vi "Vision Processing.vi"(7 "Image Size":T1=enum."320x240", 11 "error in":errorcluster) -> (4 "Sorted Scores":T6(array[cluster]) {"Correlation" format="%#_3g"; "Scale %" format="%#_3g"; "Score" format="%#_3g"}, 6 "Detected Totes":T7(array[cluster]) {"Normalized Rect"."Numeric 5" format="%#_2g"; "Normalized Rect"."Numeric 3" format="%#_2g"; "Normalized Rect"."Numeric 2" format="%#_2g"; "Normalized Rect"."Numeric" format="%#_2g"}, 8 "Particles":i32, 10 "ms to process":u32, 15 "error out":errorcluster)   [LabVIEW 2014]
doc: "This VI runs in parallel to other tasks. It gets images from the camera, processes them for color or shape and use that information to affect robot behavior."
uses:
  <vilib>/Rock Robotics/WPI/Camera/WPI_CameraSettings Read MJPG.ctl
  <vilib>/Rock Robotics/WPI/Camera/WPI_CameraImageSize.ctl
  2015-Vision/Vision/Users/Jarren/Desktop/Vision Support Code/Camera Types.ctl
  <vilib>/vision/Pattern Matching.llb/IMAQ Match Range Setting.ctl
  <vilib>/vision/Pattern Matching.llb/IMAQ Curve Parameters.ctl
  <vilib>/vision/NI_Vision_Development_Module.lvlib
panel:
  out "error out 2":errorcluster
  in  "Image Size 2":T1=enum."320x240"
  in  "error in 2":errorcluster
  out "Masked 2":T2(plugin-control)
  in  "Tote Color 2":T3={"Hue"={23.67058792990901, 48.923317529462665}, "Sat"={66.78571428571429, 255.0}, "Val"={48.571428571428584, 255.0}} {"Hue" scale=0.0..255.0 scale format="%#_3g"}
  out "Particles 2":i32
  out "ms to process 2":u32
  in  "Source 2":enum32{"Files", "Camera"}(tab)
  in  "Images 2":i32(listbox)
  in  "Folder Location 2":path=path "Sample Images/KicoffFilmingVision"
  in  "Camera Settings 2":T4={"fps"=20, "compression"=30, "Image Size"=enum."320x240"}
  in  "Camera Address 2":string="USB 1"
  in  "image files 2":string[](array[string])
  in  "Image Path 2":path=path "Sample Images/KicoffFilmingVision"
  in  "Camera Type 2":T5=enum."MS HD3000 square"
  out "Original Image 2":T2(plugin-control)
  out "Template 2":T2(plugin-control)
  out "Sorted Scores 2":T6(array[cluster]) {"Correlation" format="%#_3g"; "Scale %" format="%#_3g"; "Score" format="%#_3g"}
  in  "Annotate 2":bool=TRUE
  in  "Score Threshold 2":dbl=75.0
  out "Detected Totes 2":T7(array[cluster]) {"Normalized Rect"."Numeric 5" format="%#_2g"; "Normalized Rect"."Numeric 3" format="%#_2g"; "Normalized Rect"."Numeric 2" format="%#_2g"; "Normalized Rect"."Numeric" format="%#_2g"}
  out "Template":T2(plugin-control)
  in  "Camera Type":T5=enum."MS HD3000 square"
  in  "Image Path":path=path "Sample Images/KicoffFilmingVision"
  in  "image files":string[](array[string])
  in  "Score Threshold":dbl=75.0
  in  "Source":enum32{"Files", "Camera"}(tab)
  in  "Images":i32(listbox)
  in  "Folder Location":path=path "Sample Images/KicoffFilmingVision"
  in  "Camera Settings":T4={"fps"=20, "compression"=30, "Image Size"=enum."320x240"}
  in  "Camera Address":string="USB 1"
  in  "Annotate":bool=TRUE
  in  "Tote Color":T3={"Hue"={23.67058792990901, 48.923317529462665}, "Sat"={66.78571428571429, 255.0}, "Val"={48.571428571428584, 255.0}} {"Hue" scale=0.0..255.0 scale format="%#_3g"}
  out "Masked":T2(plugin-control)
  out "Original Image":T2(plugin-control)
  # "Instructions:\nUse Source to select image files from a directory or use a USB or IP camera connected to your laptop.\nUse Tote Color for initial processing, then search for the trained template image. Use Vision Assistant\nto train for different images or to modify Range Settings. \nThis example is effective within a few feet. It is likely not the right choice for distant patterns.\nAnnotations show the rectangle and the scores from top to bottom."
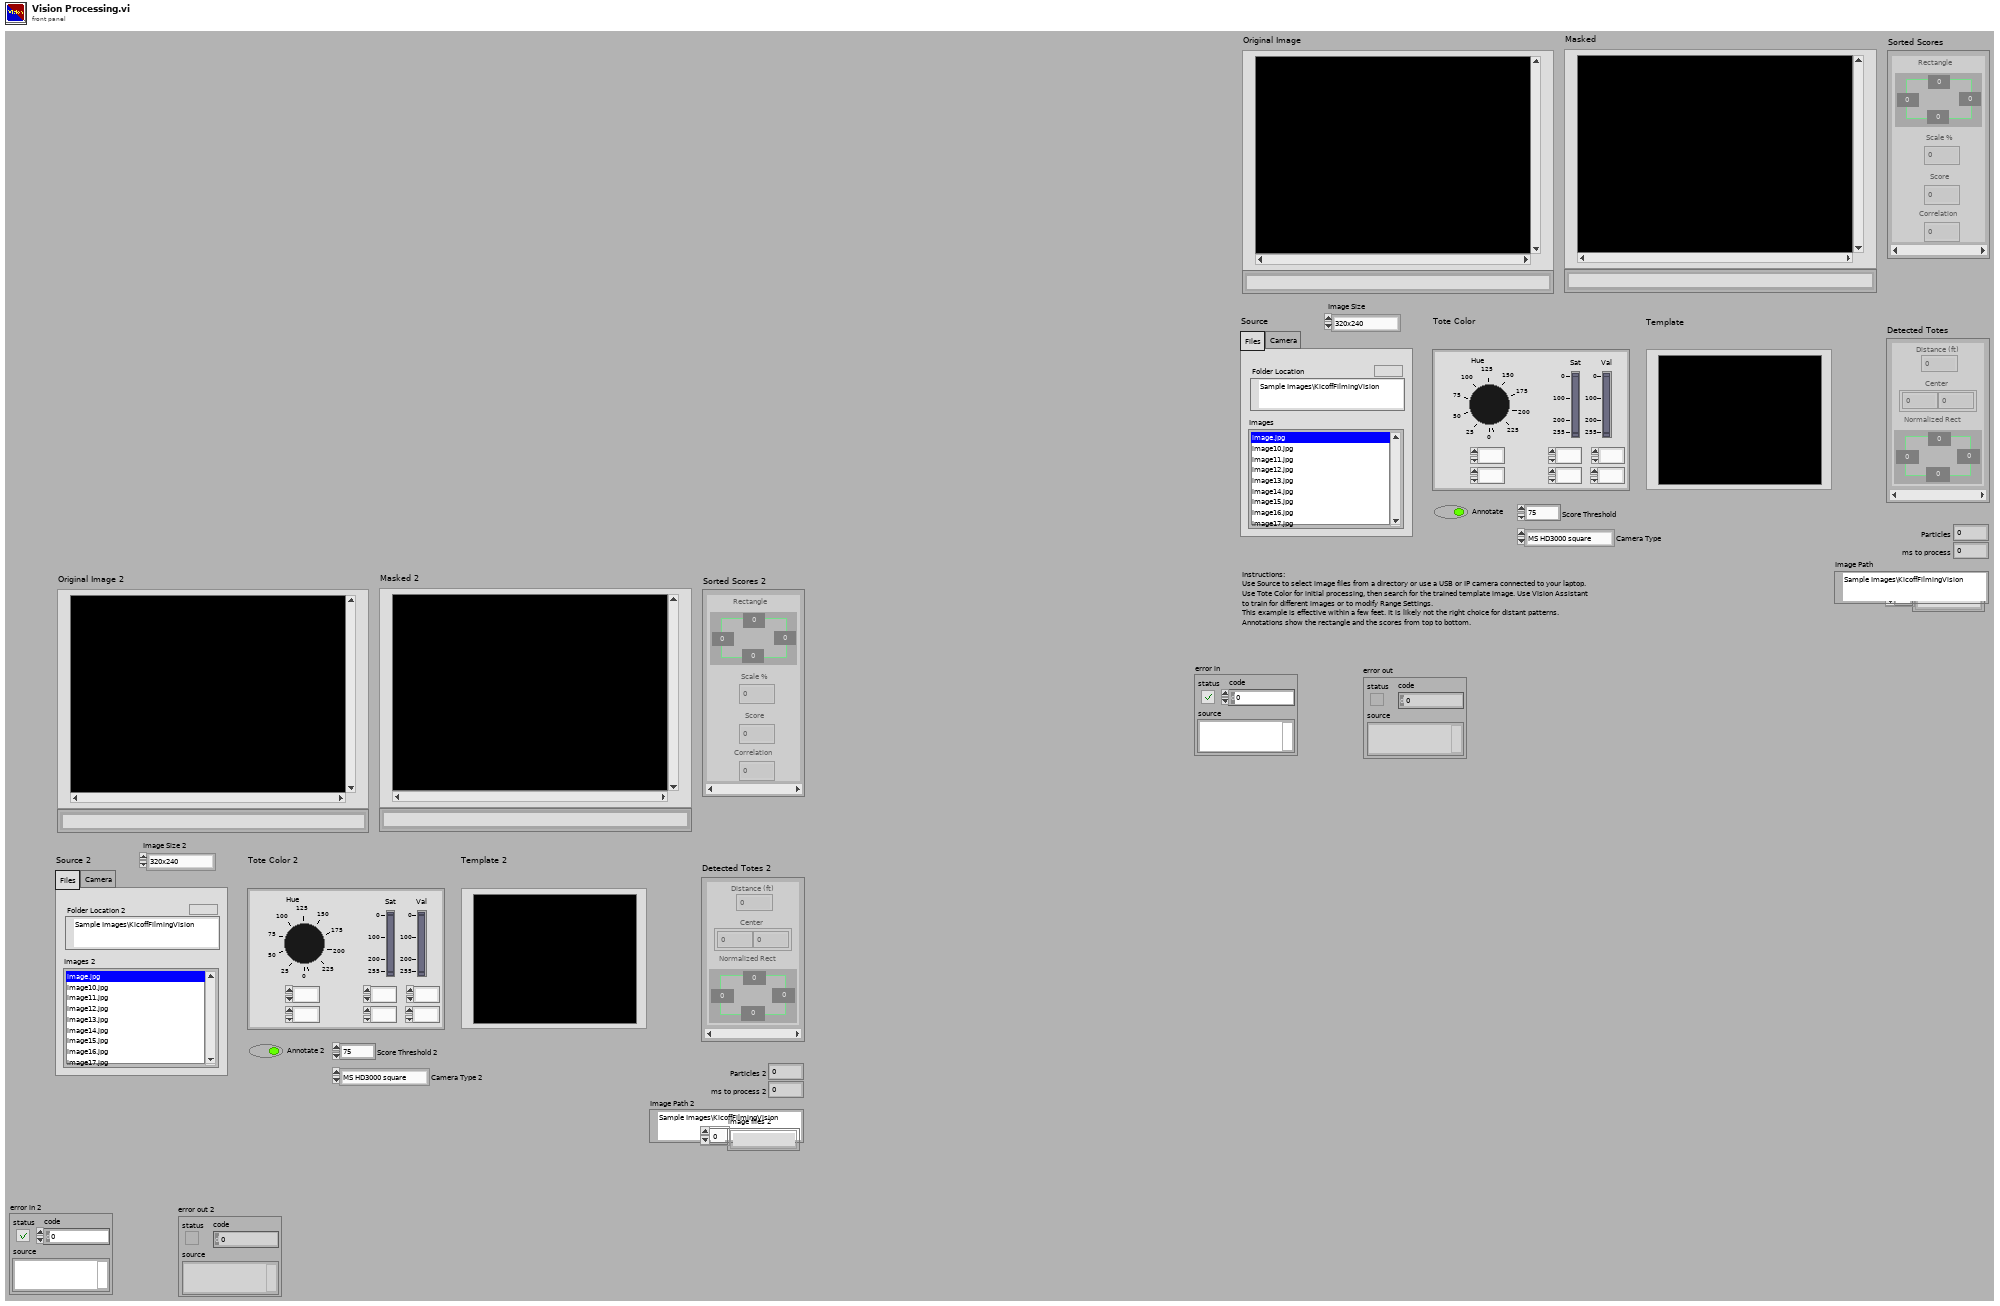
[diagram p1: front panel]
types:
  T1 = typedef "WPI_CameraImageSize.ctl" = enum16{"640x480", "320x240", "160x120", "Custom"}
  T2 = typedef "IMAQ Image.ctl" = refnum<image>
  T3 = cluster{"Hue":cluster{dbl, dbl}, "Sat":cluster{dbl, dbl}, "Val":cluster{dbl, dbl}}
  T4 = typedef "WPI_CameraSettings Read MJPG.ctl" = cluster{"fps":i32, "compression":i32, "Image Size":T1}
  T5 = typedef "Camera Types.ctl" = enum16{"206", "1011", "1013", "MS HD3000 square", "MS HD3000 640x480"}
  T6 = cluster{"Rectangle":cluster{"Numeric":dbl, "Numeric 2":dbl, "Numeric 3":dbl, "Numeric 5":dbl}, "Scale %":dbl, "Score":dbl, "Correlation":dbl}[]
  T7 = cluster{"Distance (ft)":dbl, "Center":cluster{dbl, dbl}, "Normalized Rect":cluster{"Numeric":dbl, "Numeric 2":dbl, "Numeric 3":dbl, "Numeric 5":dbl}}[]
  T8 = cluster{"Rotation":bool, "Scale":bool, "Occlusion":bool, "Reserved":bool, "Reserved":bool, "Reserved":bool}
  T9 = typedef "IMAQ Curve Parameters.ctl" = cluster{"Extraction Mode":u32, "Edge Threshold":i32, "Edge Filter Size":u32, "Min Length":i32, "Row Search Step Size":i32, "Col Search Step Size":i32, "Max Endpoint Gap":i32, "Closed":bool, "Subpixel":bool}
  T10 = typedef "IMAQ Match Range Setting.ctl" = cluster{"Match Constraints":u32, "Min":dbl, "Max":dbl}
  T11 = typedef "Image Type" = u32
  T12 = typedef "Particle Parameters" = i32
  T13 = cluster{"[0]":dbl, "[1]":dbl, "[2]":dbl, "[3]":dbl}
  T14 = cluster{"[0]":dbl, "[1]":dbl, "[2]":dbl, "[3]":dbl, "[4]":dbl}
  T15 = typedef "ROI Descriptor" = cluster{"Global Rectangle":i32[], "Contours":cluster{"ID":enum32{"External", "Internal"}, "Type":u32, "Coordinates":i32[]}[]}
  T16 = typedef "IMAQ GM Match Report.ctl" = cluster{"Position":cluster{"x":sgl, "y":sgl}, "Angle":sgl, "Scale":sgl, "Score":sgl, "Bounding Box":cluster{"x":sgl, "y":sgl}[], "Contrast Reversed":bool, "Occlusion %":sgl, "Template Target Curve Score":sgl, "Target Template Curve Score":sgl, "Correlation Score":sgl}
  T17 = cluster{cluster{"[0]":dbl, "[1]":dbl, "[2]":dbl, "[3]":dbl}, "Position":cluster{"x":sgl, "y":sgl}, "Bounding Box":cluster{"x":sgl, "y":sgl}[], "Scale":sgl, "Score":sgl, "Correlation Score":sgl}
  T18 = cluster{"Rectangle":cluster{"Numeric":dbl, "Numeric 2":dbl, "Numeric 3":dbl, "Numeric 5":dbl}, "Scale":dbl, "Score":dbl, "Correlation":dbl}[]
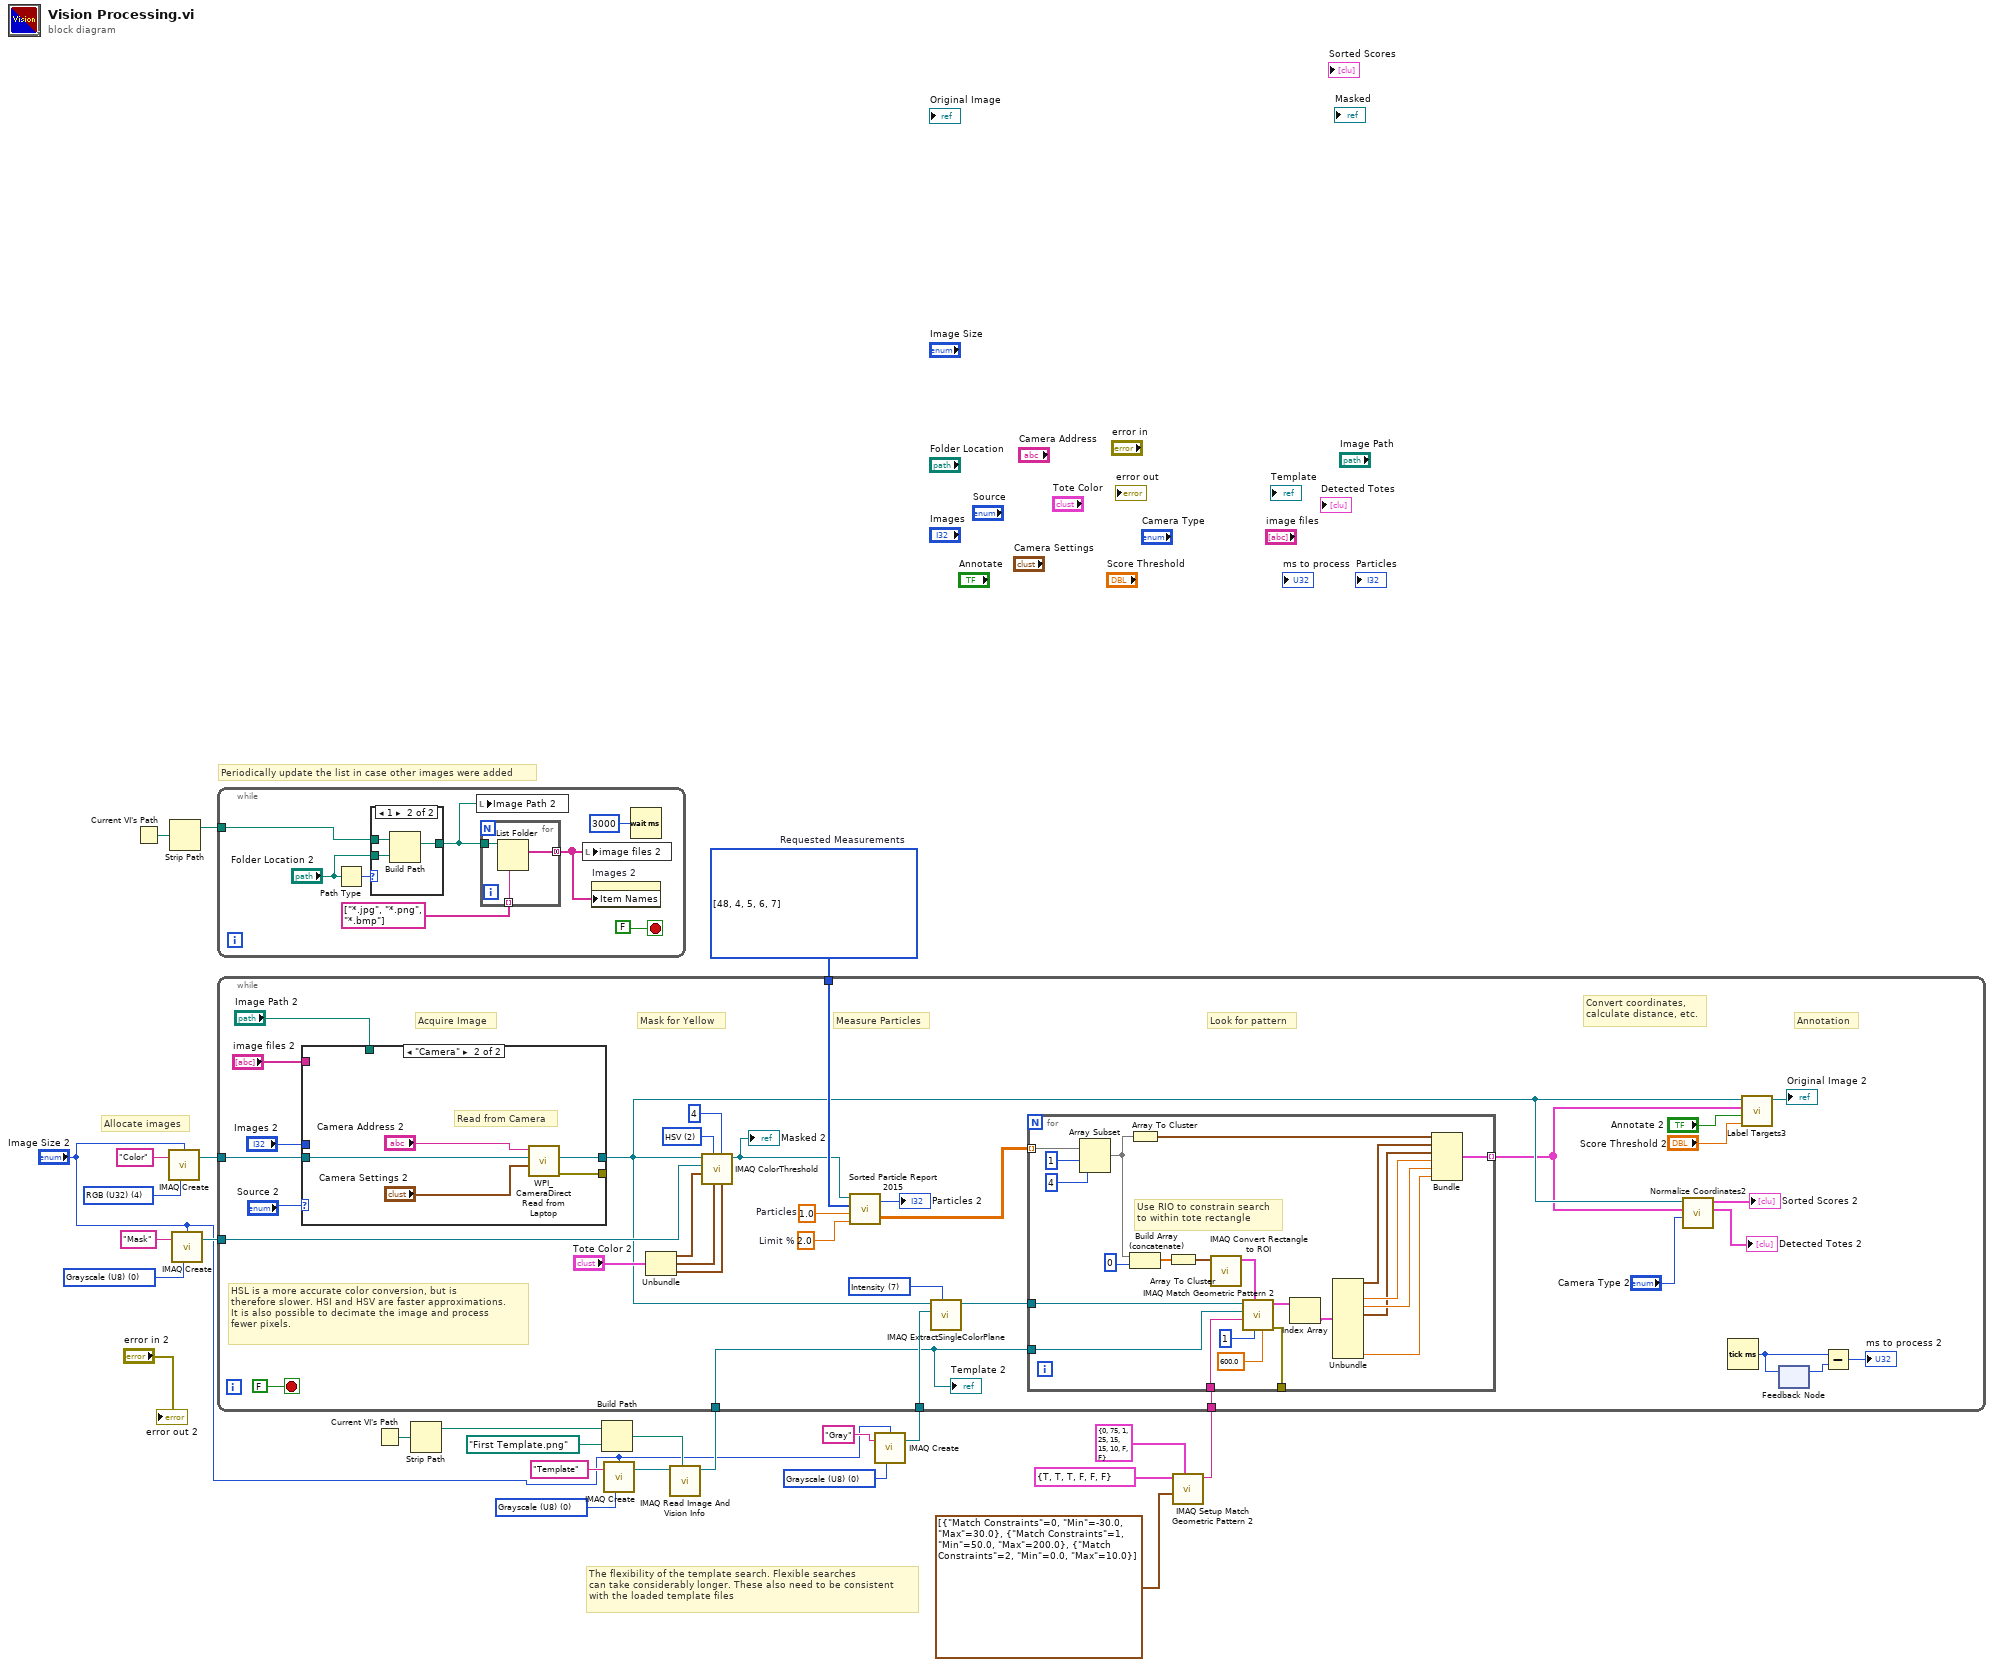
[diagram p0: block diagram]
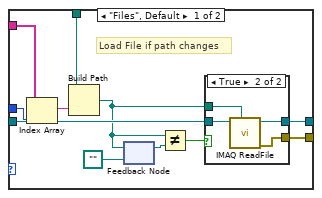
[diagram p3: hidden frame]
diagram:
  w15 = T11 0 items=["Grayscale (U8)", "Grayscale (I16)", "Grayscale (SGL)", "Complex (CSG)", "RGB (U32)", "HSL (U32)", "RGB (U64)", "Grayscale (U16)"] ("Image Type")
  w17 = T11 0 items=["Grayscale (U8)", "Grayscale (I16)", "Grayscale (SGL)", "Complex (CSG)", "RGB (U32)", "HSL (U32)", "RGB (U64)", "Grayscale (U16)"] ("Image Type")
  w20 = T12[] [48, 4, 5, 6, 7] items=["Center of Mass X", "Center of Mass Y", "First Pixel X", "First Pixel Y", "Bounding Rect Left", "Bounding Rect Top", "Bounding Rect Right", "Bounding Rect Bottom", "Max Feret Diameter Start X", "Max Feret Diameter Start Y", "Max Feret Diameter End X", "Max Feret Diameter End Y", "Max Horiz. Segment Length Left", "Max Horiz. Segment Length Right", "Max Horiz. Segment Length Row", "-", "Bounding Rect Width", "Bounding Rect Height", "Bounding Rect Diagonal", "Perimeter", "Convex Hull Perimeter", "Holes' Perimeter", "Max Feret Diameter", "Equivalent Ellipse Major Axis", "Equivalent Ellipse Minor Axis", "Equivalent Ellipse Minor Axis (Feret)", "Equivalent Rect Long Side", "Equivalent Rect Short Side", "Equivalent Rect Diagonal", "Equivalent Rect Short Side (Feret)", "Average Horiz. Segment Length", "Average Vert. Segment Length", "Hydraulic Radius", "Waddel Disk Diameter", "-", "Area", "Holes' Area", "Particle & Holes' Area", "Convex Hull Area", "Image Area", "-", "Number of Holes", "Number of Horiz. Segments", "Number of Vert. Segments", "-", "Orientation", "Max Feret Diameter Orientation", "-", "% Area/Image Area", "% Area/(Particle & Holes' Area)", "Ratio of Equivalent Ellipse Axes", "Ratio of Equivalent Rect Sides", "-", "Elongation Factor", "Compactness Factor", "Heywood Circularity Factor", "Type Factor", "-", "Sum X", "Sum Y", "Sum XX", "Sum XY", "Sum YY", "Sum XXX", "Sum XXY", "Sum XYY", "Sum YYY", "-", "Moment of Inertia XX", "Moment of Inertia XY", "Moment of Inertia YY", "Moment of Inertia XXX", "Moment of Inertia XXY", "Moment of Inertia XYY", "Moment of Inertia YYY", "Norm. Moment of Inertia XX", "Norm. Moment of Inertia XY", "Norm. Moment of Inertia YY", "Norm. Moment of Inertia XXX", "Norm. Moment of Inertia XXY", "Norm. Moment of Inertia XYY", "Norm. Moment of Inertia YYY", "Hu Moment 1", "Hu Moment 2", "Hu Moment 3", "Hu Moment 4", "Hu Moment 5", "Hu Moment 6", "Hu Moment 7"]  # Requested Measurements
  w23 = T11 0 items=["Grayscale (U8)", "Grayscale (I16)", "Grayscale (SGL)", "Complex (CSG)", "RGB (U32)", "HSL (U32)", "RGB (U64)", "Grayscale (U16)"] ("Image Type")
  w25 = T11 4 items=["Grayscale (U8)", "Grayscale (I16)", "Grayscale (SGL)", "Complex (CSG)", "RGB (U32)", "HSL (U32)", "RGB (U64)", "Grayscale (U16)"] ("Image Type")
  # "The flexibility of the template search. Flexible searches\ncan take considerably longer. These also need to be consistent\nwith the loaded template files"
  # "Periodically update the list in case other images were added"
  # "Allocate images"
  n1 = Current VI's Path() -> (path=w19:path)
  n2 = call "IMAQ Create"("Border Size"="Image Size 2", "Image Name"="Color", "Image Type"=w25) -> ("New Image"=w24:T2)  [unwired: 1 in, 2 out]
  n3 = Strip Path(path=w19) -> (stripped path=w18:path)  [unwired: 1 out]
  n4 = call "IMAQ Create"("Border Size"="Image Size 2", "Image Name"="Mask", "Image Type"=w23) -> ("New Image"=w21:T2)  [unwired: 1 in, 2 out]
  n5 = while {
    tunnel: w18 -> [w28]
    stop <- FALSE stop-if-true
    n6 = Path Type(1:"Folder Location 2") -> (0:w30:i16)
    n7 = case shown="1" w30 {
      tunnel: "Folder Location 2" -> [w35 w38]
      tunnel: [w35 w36] -> w27
      tunnel: w28 -> [_ w37]
      frame 0, Default {
      }
      frame 1 {
        n8 = Build Path(base path=w37, name or relative path=w38) -> (appended path=w36:path)
      }
    }
    n9 = local write "Image Path 2"(w27) -> ()
    n10 = for {
      tunnel: [w41] -> w31 mode=concatenating
      tunnel: w27 -> [w40]
      tunnel: string[] ["*.jpg", "*.png", "*.bmp"] -> [w39] mode=indexing
      n11 = List Folder(path=w40, pattern=w39) -> (filenames=w41:string[])  [unwired: 2 in, 3 out]
    }
    n12 = local write "image files 2"(w31) -> ()
    n13 = property on="Images 2" class="LstBox (strict)"("Item Names"=w31) -> ()  [unwired: 2 in, 2 out]
    n14 = Wait (ms)(milliseconds to wait=u32 3000) -> ()  [unwired: 1 out]
  }
  n15 = Current VI's Path() -> (path=w4:path)
  n16 = Strip Path(path=w4) -> (stripped path=w3:path)  [unwired: 1 out]
  n17 = Build Path(base path=w3, name or relative path=path "First Template.png") -> (appended path=w5:path)
  n18 = call "IMAQ Create"("Border Size"="Image Size 2", "Image Name"="Template", "Image Type"=w15) -> ("New Image"=w7:T2)  [unwired: 1 in, 2 out]
  n19 = call "IMAQ Read Image And Vision Info"("File Path"=w5, "Image"=w7) -> ("Image Out"=w6:T2)  [unwired: 2 in, 7 out]
  n20 = call "IMAQ Create"("Border Size"="Image Size 2", "Image Name"="Gray", "Image Type"=w17) -> ("New Image"=w9:T2)  [unwired: 1 in, 2 out]
  n21 = call "IMAQ Setup Match Geometric Pattern 2"("Curve Parameters"=T9 {"Extraction Mode"=0, "Edge Threshold"=75, "Edge Filter Size"=1, "Min Length"=25, "Row Search Step Size"=15, "Col Search Step Size"=15, "Max Endpoint Gap"=10, "Closed"=FALSE, "Subpixel"=FALSE}, "Range Settings"=T10[] [{"Match Constraints"=0, "Min"=-30.0, "Max"=30.0}, {"Match Constraints"=1, "Min"=50.0, "Max"=200.0}, {"Match Constraints"=2, "Min"=0.0, "Max"=10.0}], "Match Mode"=T8 {"Rotation"=TRUE, "Scale"=TRUE, "Occlusion"=TRUE, "Reserved"=FALSE, "Reserved"=FALSE, "Reserved"=FALSE}) -> ("Match Geometric Pattern 2 Setup Data"=w10:string)  [unwired: 7 in, 1 out]
  n22 = while {
    tunnel: w24 -> [w75]
    tunnel: w21 -> [w73]
    tunnel: w20 -> [w67]
    tunnel: w10 -> [w54]
    tunnel: w9 -> [w52]
    tunnel: w6 -> [w42]
    stop <- FALSE stop-if-true
    w56 = 7 items=["Red", "Green", "Blue", "Hue", "Saturation", "Luminance", "Value", "Intensity"] ("Color Plane")
    w64 = 2.0  # Limit %
    w66 = 1.0  # Particles
    w72 = u16 2 items=["RGB", "HSL", "HSV", "HSI"] ("Color Mode")
    # "Convert coordinates,\ncalculate distance, etc."
    # "Annotation"
    # "Measure Particles"
    # "Look for pattern"
    # "Mask for Yellow"
    # "Acquire Image"
    # "HSL is a more accurate color conversion, but is\ntherefore slower. HSI and HSV are faster approximations.\nIt is also possible to decimate the image and process\nfewer pixels."
    n23 = case shown="\"Camera\"" "Source 2" {
      tunnel: [w109 w120] -> _
      tunnel: [w110 w119] -> w47
      tunnel: w75 -> [w108 w118]
      tunnel: "image files 2" -> [w100 _]
      tunnel: "Images 2" -> [w107 _]
      tunnel: "Image Path 2" -> [w105 _]
      frame "Files", Default {
        # "Load File if path changes"
        n24 = Index Array(array=w100, index=w107) -> (element=w106:string)
        n25 = Build Path(base path=w105, name or relative path=w106) -> (appended path=w101:path)
        n26 = feedback-in #1(w101) -> ()
        n27 = feedback #1(path "" ("appended path")) -> (w103:path)
        n28 = Not Equal?(x=w101, y=w103) -> (x != y?=w104:bool)
        n29 = case shown="True" w104 {
          tunnel: [w111 w115] -> w110
          tunnel: [_ w114] -> w109
          tunnel: w108 -> [w111 w113]
          tunnel: w101 -> [_ w112]
          frame False {
          }
          frame True {
            n30 = call "IMAQ ReadFile"("File Path"=w112, "Image"=w113) -> ("error out"=w114:errorcluster, "Image Out"=w115:T2)  [unwired: 5 in, 3 out]
          }
        }
      }
      frame "Camera" {
        # "Read from Camera"
        n31 = call <vilib>:"WPI_CameraDirect Read from Laptop.vi"("Camera Settings"="Camera Settings 2", "Image"=w118, "address"="Camera Address 2") -> ("error out"=w120:errorcluster, "Image Out"=w119:T2)  [unwired: 7 in]
      }
    }
    n32 = Unbundle("Tote Color 2") -> ("Hue"=w71:cluster{dbl, dbl}, "Sat"=w70:cluster{dbl, dbl}, "Val"=w69:cluster{dbl, dbl})
    n33 = call "IMAQ ColorThreshold"("Blue or Luma or Val or Inten Range"=w69, "Replace Value"=4, "Green or Sat Range"=w70, "Color Mode"=w72, "Red or Hue Range"=w71, "Image Dst"=w73, "Image Src"=w47) -> ("Image Dst Out"=w55:T2)  [unwired: 3 in, 1 out]
    "Masked 2" <- w55
    n34 = call "Sorted Particle Report 2015.vi"("Min Area Size %"=w64, "Particle Count Limit"=w66, "Pixel Measurements"=w67, "Image in"=w55) -> ("Sorted Data"=w51:dbl[][], "Particles"=→"Particles 2":i32)
    n35 = call "IMAQ ExtractSingleColorPlane"("Color Plane"=w56, "Image Dst"=w52, "Image Src"=w47) -> ("Image Dst Out"=w53:T2)  [unwired: 7 in, 1 out]
    n36 = for {
      tunnel: w51 -> [w97] mode=indexing
      tunnel: [w96] -> w46 mode=indexing
      tunnel: w53 -> [w87]
      tunnel: w54 -> [w89]
      tunnel: w42 -> [w79]
      tunnel: [w78] -> _
      # "Use RIO to constrain search\nto within tote rectangle"
      n37 = Array Subset(array=w97, index=1, length=4) -> (w90:dbl[])
      n38 = Array To Cluster(array=w90) -> (cluster=w91:T13)
      n39 = Build Array (concatenate)(w90, 0 ("length")) -> (w94:dbl[])
      n40 = Array To Cluster(array=w94) -> (cluster=w93:T14)
      n41 = call "IMAQ Convert Rectangle to ROI"("Rectangle"=w93) -> ("ROI Descriptor"=w92:T15)  [unwired: 8 in, 1 out]
      n42 = call "IMAQ Match Geometric Pattern 2"("Minimum Match Score"=sgl 600.0, "Number of Matches Requested"=1 ("Minimum Match Score"), "ROI Descriptor"=w92, "Match Geometric Pattern 2 Setup Data"=w89, "Template Image"=w79, "Image"=w87) -> ("error out"=w78:errorcluster, "Matches (pixel)"=w85:T16[])  [unwired: 2 in, 2 out]
      n43 = Index Array(array=w85) -> (element=w84:T16)  [unwired: 1 in]
      n44 = Unbundle(w84) -> ("Position"=w83:cluster{"x":sgl, "y":sgl}, "Scale"=w82:sgl, "Score"=w81:sgl, "Bounding Box"=w77:cluster{"x":sgl, "y":sgl}[], "Correlation Score"=w80:sgl)  [unwired: 5 out]
      n45 = Bundle(w91, "Position"=w83, "Bounding Box"=w77, "Scale"=w82, "Score"=w81, "Correlation Score"=w80) -> (w96:T17)  [unwired: 1 in]
    }
    n46 = call "Normalize Coordinates2.vi"("Camera Type"="Camera Type 2", "Targets"=w46, "Image in"=w47) -> ("Found Totes"=→"Detected Totes 2":T7, "Sorted Scores"=→"Sorted Scores 2":T18)  [unwired: 7 in]
    n47 = Tick Count (ms)() -> (millisecond timer value=w62:u32)
    n48 = call "Label Targets3.vi"("Score Threshold"="Score Threshold 2", "Annotate"="Annotate 2", "Targets"=w46, "Image in"=w47) -> ("Image out"=→"Original Image 2":T2)  [unwired: 7 in]
    n49 = feedback-in #2(w62) -> ()
    n50 = feedback #2() -> (w63:u32)  [unwired: 1 in]
    n51 = Subtract(x=w62, y=w63) -> (x-y=→"ms to process 2":u32)
    "Template 2" <- w42
  }
  "error out 2" <- "error in 2"
